vi "Stop-DetectorSD.vi"() -> (0 "Stopped":bool)   [LabVIEW 2015]
uses:
  globalVarSD.vi
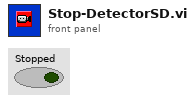
[diagram p1: front panel]
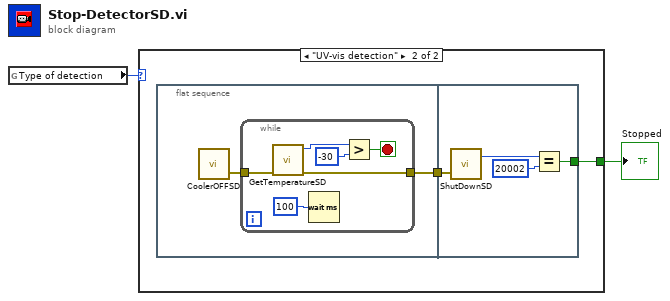
[diagram p0: block diagram]
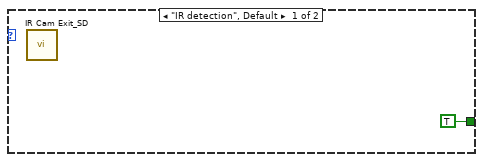
[diagram p2: hidden frame]
diagram:
  n1 = global read "globalVarSD.vi" "Type of detection"() -> (w1:enum32{"IR detection", "UV-vis detection"})
  n2 = case shown="\"UV-vis detection\"" w1 {
    tunnel: [TRUE w4] -> w2
    frame "IR detection", Default {
      n3 = call "IR Cam Exit_SD.vi"() -> ()  [unwired: 1 in]
    }
    frame "UV-vis detection" {
      n4 = flat-sequence {
        tunnel: [w6] -> w5
        tunnel: [w15] -> w4
        tunnel: w5 -> [w14]
        frame #0 {
          n5 = call "CoolerOFFSD.vi"() -> ("error out"=w7:errorcluster)  [unwired: 2 in, 1 out]
          n6 = while {
            tunnel: w7 -> [w13]
            tunnel: [w8] -> w6
            stop <- w11 stop-if-true
            n7 = call "GetTemperatureSD.vi"("error in (no error)"=w13) -> ("error out"=w8:errorcluster, "temperature"=w10:i32)  [unwired: 3 in, 2 out]
            n8 = Wait (ms)(milliseconds to wait=u32 100) -> ()  [unwired: 1 out]
            n9 = Greater?(x=w10, y=-30) -> (0:w11:bool)
          }
        }
        frame #1 {
          n10 = call "ShutDownSD.vi"("error in (no error)"=w14) -> ("DLL error code"=w16:u32)  [unwired: 1 in, 1 out]
          n11 = Equal?(x=w16, y=u32 20002) -> (x = y?=w15:bool)
        }
      }
    }
  }
  "Stopped" <- w2
